vi "UpdateSetMembership.vi"(10 "node ref in":refnum<data-value>, 11 "RVCLibrary_Bug in":refnum<class "RVCLibrary_Bug2.lvclass">) -> (2 "node ref out":refnum<data-value>, 3 "RVCLibrary_Bug out":refnum<class "RVCLibrary_Bug2.lvclass">)   [LabVIEW 2013, in "RVCLibrary_Bug2.lvclass"]
uses:
  RVCLibrary_Bug2.lvclass
  <vilib>/robotics/Navigation/shared/MapNode/AbstractDstarNode/NI_Robotics_AbstractDstarNode.lvclass
  RVCLibrary_Bug2.lvclass/RVCLibrary_Bug2.ctl
  <vilib>/robotics/Navigation/shared/Priority Queue/NI_Robotics_Priority Queue.lvclass
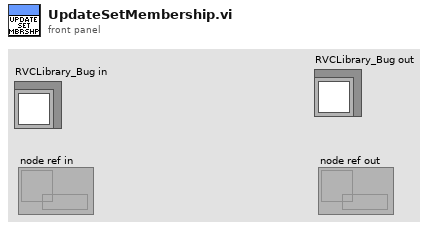
[diagram p1: front panel]
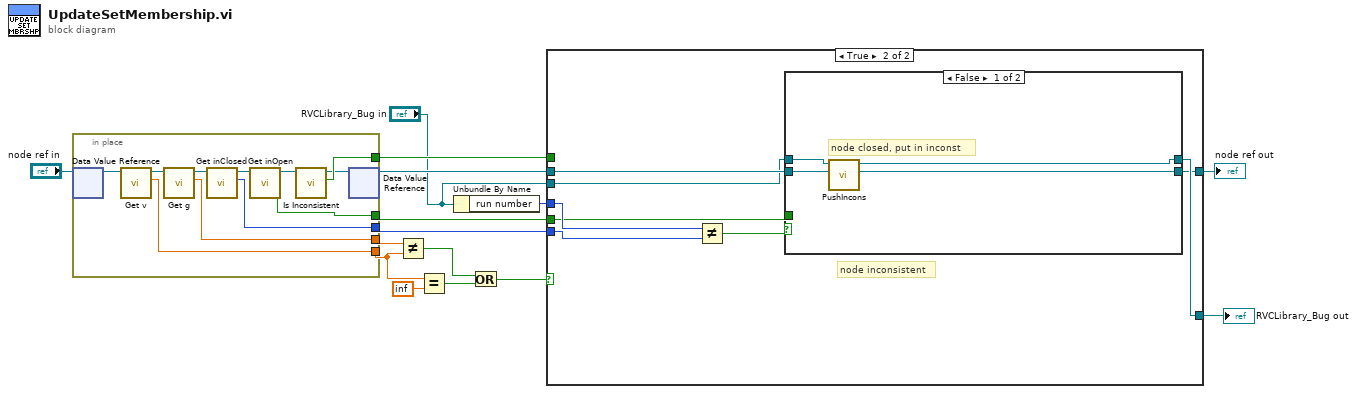
[diagram p0: block diagram]
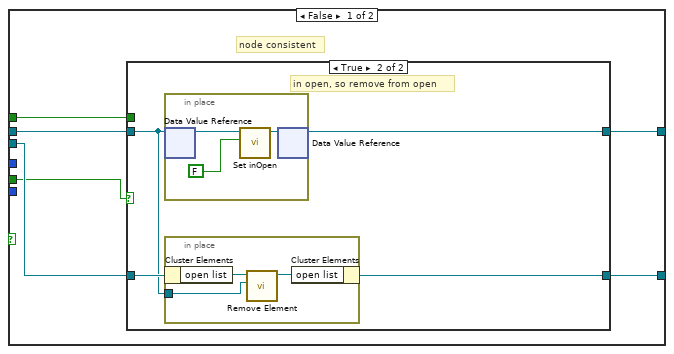
[diagram p2: hidden frame]
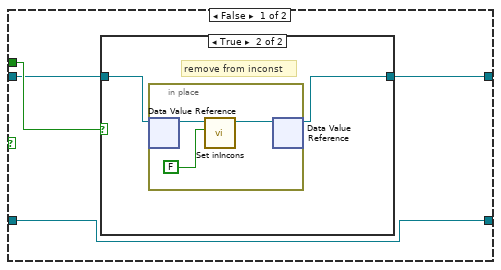
[diagram p3: hidden frame]
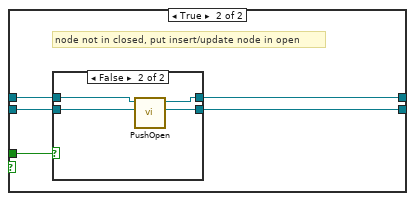
[diagram p5: hidden frame]
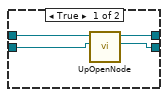
[diagram p6: hidden frame]
diagram:
  n1 = in-place {
    in-place-border: [w23] -> w14
    in-place-border: [w22] -> w6
    in-place-border: [w21] -> w5
    in-place-border: [w19] -> w4
    in-place-border: [w17] -> w3
    n2 = in-place-dvr #1("node ref in") -> (w26:refnum<class "NI_Robotics_AbstractDstarNode.lvclass">)  [unwired: 1 out]
    n3 = call <vilib>:"Get v.vi"("AbstractDstarNode in"=w26) -> ("v"=w21:dbl, "AbstractDstarNode out"=w25:refnum<class "NI_Robotics_AbstractDstarNode.lvclass">)  [unwired: 9 in]
    n4 = call <vilib>:"Get g.vi"("AbstractDstarNode in"=w25) -> ("g"=w22:dbl, "AbstractDstarNode out"=w24:refnum<class "NI_Robotics_AbstractDstarNode.lvclass">)  [unwired: 9 in]
    n5 = call <vilib>:"Get inClosed.vi"("AbstractDstarNode in"=w24) -> ("inClosed"=w23:i32, "AbstractDstarNode out"=w20:refnum<class "NI_Robotics_AbstractDstarNode.lvclass">)  [unwired: 8 in, 1 out]
    n6 = call <vilib>:"Get inOpen.vi"("AbstractDstarNode in"=w20) -> ("inOpen"=w19:bool, "AbstractDstarNode out"=w18:refnum<class "NI_Robotics_AbstractDstarNode.lvclass">)  [unwired: 8 in, 1 out]
    n7 = call <vilib>:"Is Inconsistent.vi"("AbstractDstarNode in"=w18) -> ("is Inconsistent"=w17:bool, "AbstractDstarNode out"=w16:refnum<class "NI_Robotics_AbstractDstarNode.lvclass">)  [unwired: 8 in, 1 out]
    n8 = in-place-dvr #1(w16) -> (w12:refnum<data-value>)  [unwired: 1 out]
  }
  n9 = Not Equal?(x=w6, y=w5) -> (x != y?=w10:bool)
  n10 = Equal?(x=w5, y=inf) -> (x = y?=w8:bool)
  n11 = Unbundle By Name("RVCLibrary_Bug in") -> ("run number"=w13:i32)
  n12 = Or(x=w10, y=w8) -> (x .or. y?=w9:bool)
  n13 = case shown="True" w9 {
    tunnel: [w30 w59] -> w1
    tunnel: w14 -> [_ w58]
    tunnel: w13 -> [_ w57]
    tunnel: w12 -> [w29 w56]
    tunnel: "RVCLibrary_Bug in" -> [w31 w55]
    tunnel: [w32 w54] -> w11
    tunnel: w4 -> [w28 w53]
    tunnel: w3 -> [w27 _]
    frame False {
      # "node consistent"
      n14 = case shown="True" w28 {
        tunnel: [w33 w46] -> w32
        tunnel: w31 -> [w34 w45]
        tunnel: [w34 w44] -> w30
        tunnel: w29 -> [w35 w43]
        tunnel: w27 -> [w36 _]
        frame False {
          n15 = case shown="True" w36 {
            tunnel: w35 -> [w37 w39]
            tunnel: [w37 w38] -> w33
            frame False {
            }
            frame True {
              # "remove from inconst"
              n16 = in-place {
                n17 = in-place-dvr #2(w39) -> (w40:refnum<class "NI_Robotics_AbstractDstarNode.lvclass">)  [unwired: 1 out]
                n18 = call <vilib>:"Set inIncons.vi"("inIncons"=FALSE ("inOpen"), "AbstractDstarNode in"=w40) -> ("AbstractDstarNode out"=w42:refnum<class "NI_Robotics_AbstractDstarNode.lvclass">)  [unwired: 9 in]
                n19 = in-place-dvr #2(w42) -> (w38:refnum<data-value>)  [unwired: 1 out]
              }
            }
          }
        }
        frame True {
          # "in open, so remove from open"
          n20 = in-place {
            n21 = in-place-dvr #3(w43) -> (w50:refnum<class "NI_Robotics_AbstractDstarNode.lvclass">)  [unwired: 1 out]
            n22 = call <vilib>:"Set inOpen.vi"("inOpen"=FALSE, "AbstractDstarNode in"=w50) -> ("AbstractDstarNode out"=w52:refnum<class "NI_Robotics_AbstractDstarNode.lvclass">)  [unwired: 8 in, 1 out]
            n23 = in-place-dvr #3(w52) -> (w46:refnum<data-value>)  [unwired: 1 out]
          }
          n24 = in-place {
            in-place-border: w43 -> [w47]
            n25 = in-place-cluster #4(w45) -> ("open list"=w48:refnum<class "NI_Robotics_Priority Queue.lvclass">)
            n26 = call <vilib>:"Remove Element.vi"("node Ref"=w47, "Priority Queue in"=w48) -> ("Priority Queue out"=w49:refnum<class "NI_Robotics_Priority Queue.lvclass">)  [unwired: 8 in, 1 out]
            n27 = in-place-cluster #4("open list"=w49) -> (w44:refnum<class "RVCLibrary_Bug2.lvclass">)
          }
        }
      }
    }
    frame True {
      # "node inconsistent"
      n28 = Not Equal?(x=w57, y=w58) -> (x != y?=w60:bool)
      n29 = case shown="False" w60 {
        tunnel: [w64 w69] -> w59
        tunnel: w56 -> [w62 w68]
        tunnel: w55 -> [w63 w67]
        tunnel: [w61 w66] -> w54
        tunnel: w53 -> [_ w65]
        frame False {
          # "node closed, put in inconst"
          n30 = call "PushIncons.vi"("node ref in"=w62, "RVCLibrary_Bug in"=w63) -> ("node ref out"=w61:refnum<data-value>, "RVCLibrary_Bug out"=w64:refnum<class "RVCLibrary_Bug2.lvclass">)  [unwired: 8 in]
        }
        frame True {
          # "node not in closed, put insert/update node in open"
          n31 = case shown="False" w65 {
            tunnel: [w71 w77] -> w69
            tunnel: w68 -> [w72 w76]
            tunnel: w67 -> [w73 w75]
            tunnel: [w70 w74] -> w66
            frame True {
              n32 = call "UpOpenNode.vi"("node ref in"=w72, "RVCLibrary_Bug2 in"=w73) -> ("node ref out"=w70:refnum<data-value>, "RVCLibrary_Bug2 out"=w71:refnum<class "RVCLibrary_Bug2.lvclass">)  [unwired: 8 in]
            }
            frame False {
              n33 = call "PushOpen.vi"("node ref in"=w76, "RVCLibrary_Bug in"=w75) -> ("node ref out"=w74:refnum<data-value>, "RVCLibrary_Bug out"=w77:refnum<class "RVCLibrary_Bug2.lvclass">)  [unwired: 8 in]
            }
          }
        }
      }
    }
  }
  "node ref out" <- w11
  "RVCLibrary_Bug out" <- w1
